vi "Server send.vi"() -> ()   [LabVIEW 2016, in "数据传输系统-03.lvlib" / "自动更新.lvlib" / "TCP文件传输系统.lvlib"]
uses:
  <vilib>/Utility/miscctls.llb/LVPointTypeDef.ctl
  <vilib>/Utility/sysdir.llb/System Directory Type.ctl
  <vilib>/Averna/Notify Icon/NotifyIcon.llb/BalloonIcon.ctl
  <vilib>/Averna/Notify Icon/NotifyIcon.llb/GetSelectedItemEvent.vi
  <vilib>/Averna/Notify Icon/NotifyIcon.llb/SetVisible.vi
  <vilib>/Averna/Notify Icon/NotifyIcon.llb/SetMenuDefaultItem.vi
  <vilib>/Averna/Notify Icon/NotifyIcon.llb/SetTipText.vi
  <vilib>/Averna/Notify Icon/NotifyIcon.llb/NotifyIcon.lvclass
panel:
  in  "选项卡控件 2":enum32{"数据传输系统", "固定站系统", "环保认证"}(tab)
  in  "选项卡控件":T1(tab)
  out "TCP发送全局簇":T2
  out "文件传输的路径":path
  in  "Application":string="版本升级文档.txt"
  in  "远程端口或服务名称":u16=11235
  out "本机网络地址":string="192.168.1.250"
  out "TCP发送全局簇 2":T2
  out "文件传输的路径 2":path
  in  "Application 2":string="update.exe"
  in  "远程端口或服务名称 2":u16=11236
  out "本机网络地址 2":string="192.168.1.250"
  out "TCP发送全局簇 3":T2
  out "文件传输的路径 3":path
  in  "Application 3":string="平台数据传输系统.exe"
  in  "远程端口或服务名称 3":u16=11234
  out "本机网络地址 3":string="192.168.1.250"
  in  "选项卡控件 3":enum32{"固定站版本txt", "固定站update", "固定站exe"}(tab)
  in  "Application 5":string="版本升级文档.txt"
  out "TCP发送全局簇 5":T2
  out "本机网络地址 5":string="192.168.1.250"
  in  "远程端口或服务名称 5":u16=10051
  out "文件传输的路径 5":path
  out "文件传输的路径 6":path
  in  "远程端口或服务名称 6":u16=10052
  out "本机网络地址 6":string="192.168.1.250"
  out "TCP发送全局簇 6":T2
  in  "Application 6":string="update.exe"
  in  "Application 4":string="一体化水质自动监测系统.exe"
  out "TCP发送全局簇 4":T2
  out "本机网络地址 4":string="192.168.1.250"
  in  "远程端口或服务名称 4":u16=10050
  out "文件传输的路径 4":path
  in  "选项卡控件 4":enum32{"环保认证版本txt", "环保认证update", "环保认证exe"}(tab)
  in  "Application 7":string="版本升级文档.txt"
  out "TCP发送全局簇 7":T2
  out "本机网络地址 7":string="192.168.1.250"
  in  "远程端口或服务名称 7":u16=10061
  out "文件传输的路径 7":path
  out "文件传输的路径 8":path
  in  "远程端口或服务名称 8":u16=10062
  out "本机网络地址 8":string="192.168.1.250"
  out "TCP发送全局簇 8":T2
  in  "Application 8":string="update.exe"
  in  "Application 9":string="一体化微型水质监测站.exe"
  out "TCP发送全局簇 9":T2
  out "本机网络地址 9":string="192.168.1.250"
  in  "远程端口或服务名称 9":u16=10050
  out "文件传输的路径 9":path
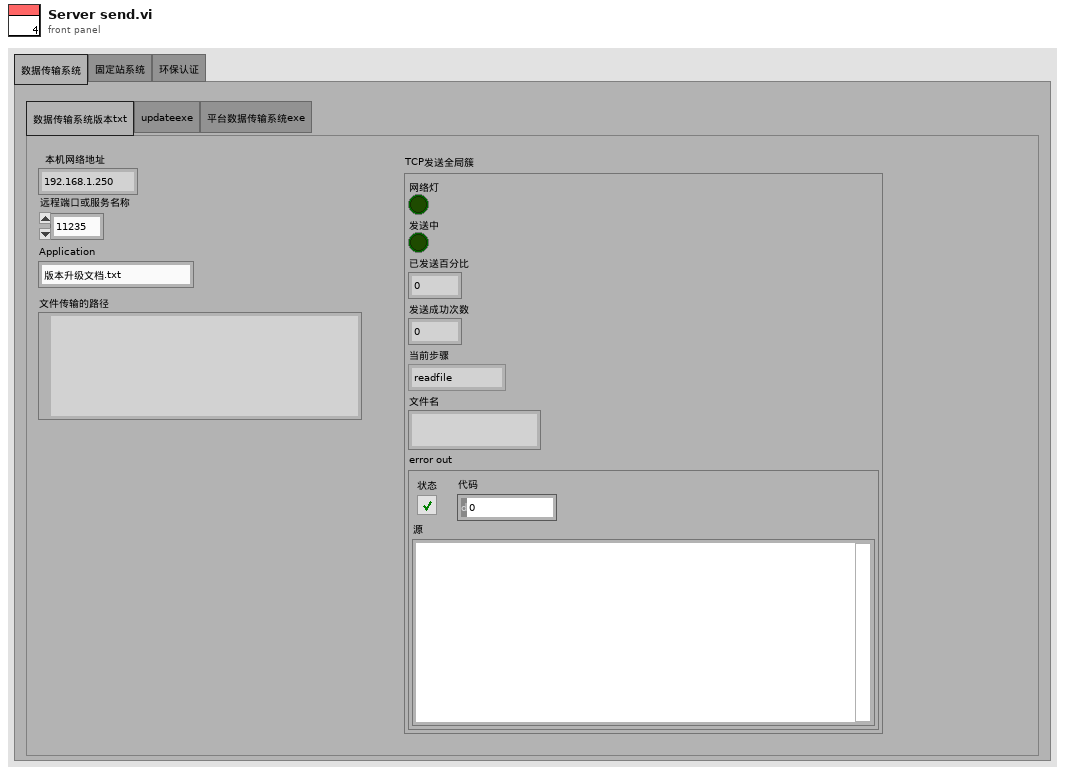
[diagram p1: front panel]
types:
  T1 = enum32{"数据传输系统版本txt", "updateexe", "平台数据传输系统exe"}
  T2 = cluster{"网络灯":bool, "发送中":bool, "已发送百分比":u8, "发送成功次数":dbl, "当前步骤":enum16{"readfile", "init", "sendhead", "sendcontent", "sendsuccess", "over"}, "文件名":string, "error out":errorcluster}
  T3 = enum32{"Invalid", "Standard", "Closed", "Hidden", "Minimized", "Maximized"}
  T4 = typedef "LVPointTypeDef.ctl" = cluster{"Horizontal":i16, "Vertical":i16}
  T5 = typedef "NotifyIcon.lvlib/NotifyIcon.lvclass/BalloonIcon.ctl" = enum32{"None", "Information", "Warning", "Error"}
  T6 = typedef "System Directory Type.ctl" = i32
  T7 = enum32{"invalid app kind", "Development System", "Run Time System", "Student Edition", "Embedded LabVIEW", "Evaluation", "Custom"}
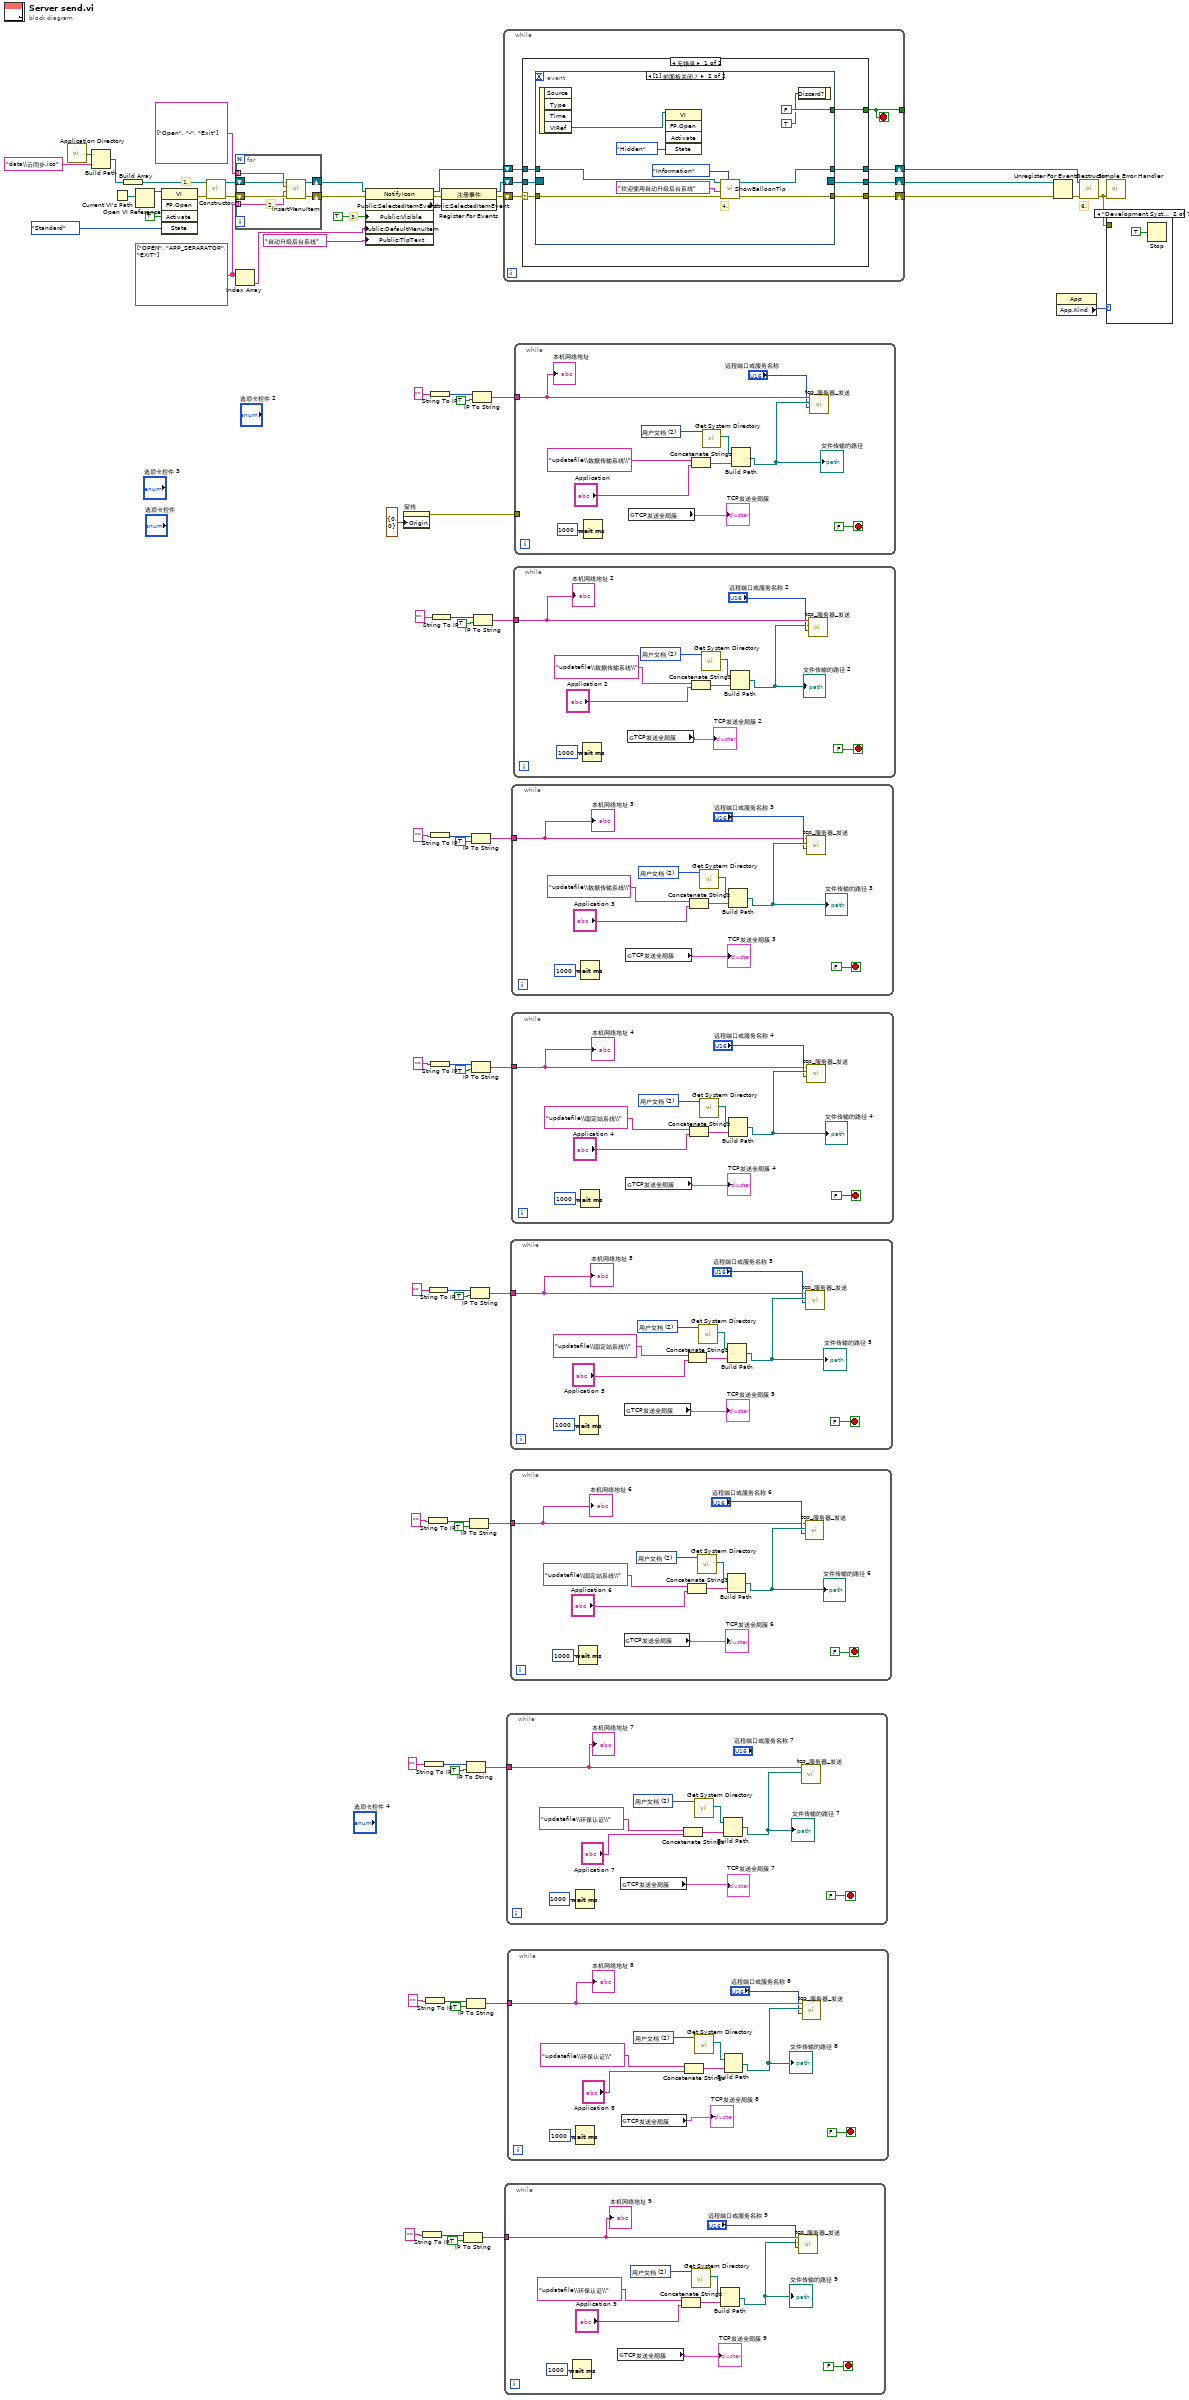
[diagram p0: block diagram]
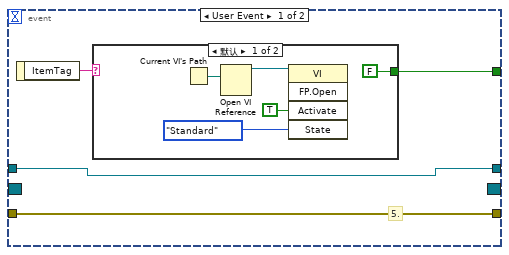
[diagram p2: hidden frame]
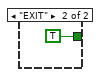
[diagram p3: hidden frame]
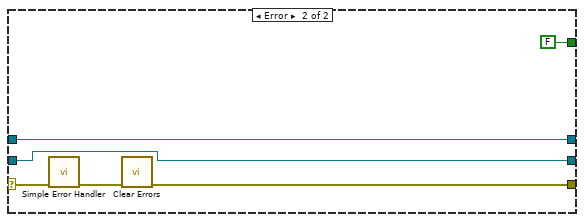
[diagram p4: hidden frame]
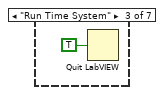
[diagram p6: hidden frame]
diagram:
  w37 = string[] ["OPEN", "APP_SEPARATOR", "EXIT"]
  # "6."
  # "3."
  # "1."
  n1 = call <vilib>:"Application Directory.vi"() -> ("Application Directory"=w35:path)
  n2 = Build Path(base path=w35, name or relative path="data\\云同步.ico" ("名称或相对路径")) -> (appended path=w45:path)
  n3 = Current VI's Path() -> (path=w32:path)
  n4 = Build Array(w45) -> (w40:path[])
  n5 = Open VI Reference(vi path=w32) -> (vi reference=w31:refnum<vi>)  [unwired: 5 in, 1 out]
  n6 = invoke class="VI" method="FP.Open"(reference=w31, "Activate"=TRUE ("激活？"), "State"=T3."Standard" ("状态")) -> (error out=w30:errorcluster)  [unwired: 2 in, 4 out]
  n7 = call <vilib>:"Constructor.vi"("error in"=w30, "IconFilePathList"=w40) -> ("error out"=w44:errorcluster, "NotifyIcon"=w36:refnum<class "NotifyIcon.lvclass">)  [unwired: 8 in]
  n8 = for {
    shift-right: [w72] -> w55
    shift-left: w44 -> [w73]
    tunnel: string[] ["Open", "-", "Exit"] -> [w71] mode=indexing
    tunnel: w37 -> [w70] mode=indexing
    shift-right: [w68] -> w54
    shift-left: w36 -> [w69]
    # "2."
    n9 = call <vilib>:"InsertMenuItem.vi"("error in"=w73, "ItemTag"=w70, "ItemName"=w71, "NotifyIcon in"=w69) -> ("error out"=w72:errorcluster, "NotifyIcon out"=w68:refnum<class "NotifyIcon.lvclass">)  [unwired: 6 in]
  }
  n10 = Index Array(array=w37) -> (element=w38:string)  [unwired: 1 in]
  n11 = property class="NotifyIcon"(reference=w54, error in=w55, "Public:Visible"=TRUE ("Visible"), "Public:DefaultMenuItem"=w38, "Public:TipText"="自动升级后台系统" ("TipText")) -> (reference out=w51:refnum<class "NotifyIcon.lvclass">, error out=w43:errorcluster, "Public:SelectedItemEvent"=w42:refnum<user-event>)
  n12 = property on="窗格" class="Pane"("Origin"=T4 {"Horizontal"=0, "Vertical"=0} ("原点")) -> (error out=w25:errorcluster)  [unwired: 2 in, 1 out]
  n13 = String To IP(1:"" ("名称")) -> (0:w2:u32)
  n14 = String To IP(1:"" ("名称")) -> (0:w10:u32)
  n15 = String To IP(1:"" ("名称")) -> (0:w6:u32)
  n16 = String To IP(1:"" ("名称")) -> (0:w14:u32)
  n17 = String To IP(1:"" ("名称")) -> (0:w19:u32)
  n18 = String To IP(1:"" ("名称")) -> (0:w58:u32)
  n19 = String To IP(1:"" ("名称")) -> (0:w22:u32)
  n20 = String To IP(1:"" ("名称")) -> (0:w65:u32)
  n21 = String To IP(1:"" ("名称")) -> (0:w61:u32)
  n22 = register-events(error in=w43, w42) -> (reference out=w27:refnum<event-registration>, error out=w28:errorcluster)  [unwired: 1 in]
  n23 = IP To String(1:TRUE ("句点符号？(F)"), 2:w2) -> (0:w1:string)
  n24 = IP To String(1:TRUE ("句点符号？(F)"), 2:w10) -> (0:w9:string)
  n25 = IP To String(1:TRUE ("句点符号？(F)"), 2:w6) -> (0:w5:string)
  n26 = IP To String(1:TRUE ("句点符号？(F)"), 2:w14) -> (0:w13:string)
  n27 = IP To String(1:TRUE ("句点符号？(F)"), 2:w19) -> (0:w20:string)
  n28 = IP To String(1:TRUE ("句点符号？(F)"), 2:w58) -> (0:w59:string)
  n29 = IP To String(1:TRUE ("句点符号？(F)"), 2:w22) -> (0:w21:string)
  n30 = IP To String(1:TRUE ("句点符号？(F)"), 2:w65) -> (0:w64:string)
  n31 = IP To String(1:TRUE ("句点符号？(F)"), 2:w61) -> (0:w60:string)
  n32 = while {
    shift-right: [w77] -> w49
    shift-left: w28 -> [w76]
    shift-right: [w78] -> w47
    shift-left: w51 -> [w79]
    shift-right: [w75] -> w48
    shift-left: w27 -> [w80]
    tunnel: [w74] -> _
    stop <- w74 stop-if-true
    n33 = case shown="无错误" w76 {
      selector: w76 -> [w82 w113]
      tunnel: w80 -> [w87 w108]
      tunnel: w79 -> [w86 w109]
      tunnel: [w85 w109] -> w78
      tunnel: [w84 w111] -> w77
      tunnel: [w83 FALSE ("Discard?")] -> w74
      tunnel: [w81 w108] -> w75
      frame No Error {
        n34 = event shown="[1] 前面板关闭？" {
          selector: w87 -> [_ _]
          dyn-events: [_ _] -> w81
          timeout: _ -> [_ _]
          tunnel: w82 -> [w90 w106]
          tunnel: [w90 w105] -> w84
          tunnel: [w89 FALSE ("Discard?")] -> w83
          tunnel: w86 -> [w88 w107]
          tunnel: [w88 w104] -> w85
          event User Event {
            # "5."
            n35 = event-data() -> ("ItemTag"=w91:string)  [unwired: 1 in]
            n36 = case shown="默认" w91 {
              tunnel: [FALSE TRUE] -> w89
              frame Default {
                n37 = Current VI's Path() -> (path=w93:path)
                n38 = Open VI Reference(vi path=w93) -> (vi reference=w94:refnum<vi>)  [unwired: 5 in, 1 out]
                n39 = invoke class="VI" method="FP.Open"(reference=w94, "Activate"=TRUE ("激活？"), "State"=T3."Standard" ("状态")) -> ()  [unwired: 2 in, 5 out]
              }
              frame "EXIT" {
              }
            }
          }
          event Panel Close? {
            # "4."
            n40 = event-data() -> ("VIRef"=w100:refnum<vi>)  [unwired: 1 in, 3 out]
            n41 = invoke class="VI" method="FP.Open"(reference=w100, "State"=T3."Hidden" ("状态")) -> ()  [unwired: 3 in, 5 out]
            n42 = call <vilib>:"ShowBalloonTip.vi"("Balloon Icon"=BalloonIcon."Information", "error in"=w106, "Text"="欢迎使用自动升级后台系统", "NotifyIcon in"=w107) -> ("error out"=w105:errorcluster, "NotifyIcon out"=w104:refnum<class "NotifyIcon.lvclass">)  [unwired: 6 in]
            n43 = event-data("Discard?"=TRUE ("放弃？")) -> ()  [unwired: 1 in, 1 out]
          }
        }
      }
      frame Error {
        n44 = call <vilib>:"Simple Error Handler.vi"("error in (no error)"=w113) -> ("error out"=w112:errorcluster)  [unwired: 4 in, 4 out]
        n45 = call <vilib>:"Clear Errors.vi"("error in (no error)"=w112) -> ("error out"=w111:errorcluster)  [unwired: 5 in, 1 out]
      }
    }
  }
  n46 = while {
    tunnel: w1 -> [w118]
    stop <- FALSE stop-if-true
    w123 = T6 2 items=["用户目录"=0, "用户桌面"=1, "用户文档"=2, "用户应用程序数据"=3, "用户设置"=4, "用户临时目录"=5, "公共文档"=6, "公共应用程序数据"=7, "公共设置"=8, "公共缓存"=13, "系统核心库"=9, "系统安装库"=10, "应用程序文件"=11, "启动盘根目录"=12] ("system directory type")
    n47 = Wait (ms)(milliseconds to wait=u32 1000 ("等待时间（毫秒）")) -> ()  [unwired: 1 out]
    n48 = global read "全局变量1.vi" "TCP发送全局簇"() -> (→"TCP发送全局簇 9":T2)
    n49 = Concatenate Strings("updatefile\\环保认证\\" ("condition"), "Application 9") -> (w122:string)
    n50 = call <vilib>:"Get System Directory.vi"("system directory type"=w123) -> ("system directory"=w121:path)  [unwired: 10 in]
    n51 = Build Path(base path=w121, name or relative path=w122) -> (appended path=w114:path)
    "文件传输的路径 9" <- w114
    n52 = call "tcp_服务器_发送.vi"("远程端口或服务名称"="远程端口或服务名称 9", "原文件路径（使用对话框）"=w114, "服务器网络地址"=w118) -> ()  [unwired: 9 in]
    "本机网络地址 9" <- w118
  }
  n53 = while {
    tunnel: w9 -> [w128]
    stop <- FALSE stop-if-true
    w133 = T6 2 items=["用户目录"=0, "用户桌面"=1, "用户文档"=2, "用户应用程序数据"=3, "用户设置"=4, "用户临时目录"=5, "公共文档"=6, "公共应用程序数据"=7, "公共设置"=8, "公共缓存"=13, "系统核心库"=9, "系统安装库"=10, "应用程序文件"=11, "启动盘根目录"=12] ("system directory type")
    n54 = Wait (ms)(milliseconds to wait=u32 1000 ("等待时间（毫秒）")) -> ()  [unwired: 1 out]
    n55 = global read "全局变量1.vi" "TCP发送全局簇"() -> (→"TCP发送全局簇 7":T2)
    n56 = Concatenate Strings("updatefile\\环保认证\\" ("condition"), "Application 7") -> (w132:string)
    n57 = call <vilib>:"Get System Directory.vi"("system directory type"=w133) -> ("system directory"=w131:path)  [unwired: 10 in]
    n58 = Build Path(base path=w131, name or relative path=w132) -> (appended path=w126:path)
    "文件传输的路径 7" <- w126
    n59 = call "tcp_服务器_发送.vi"("原文件路径（使用对话框）"=w126, "服务器网络地址"=w128) -> ()  [unwired: 10 in]
    "本机网络地址 7" <- w128
  }
  n60 = while {
    tunnel: w5 -> [w139]
    stop <- FALSE stop-if-true
    w144 = T6 2 items=["用户目录"=0, "用户桌面"=1, "用户文档"=2, "用户应用程序数据"=3, "用户设置"=4, "用户临时目录"=5, "公共文档"=6, "公共应用程序数据"=7, "公共设置"=8, "公共缓存"=13, "系统核心库"=9, "系统安装库"=10, "应用程序文件"=11, "启动盘根目录"=12] ("system directory type")
    n61 = Wait (ms)(milliseconds to wait=u32 1000 ("等待时间（毫秒）")) -> ()  [unwired: 1 out]
    n62 = global read "全局变量1.vi" "TCP发送全局簇"() -> (→"TCP发送全局簇 8":T2)
    n63 = Concatenate Strings("updatefile\\环保认证\\" ("condition"), "Application 8") -> (w143:string)
    n64 = call <vilib>:"Get System Directory.vi"("system directory type"=w144) -> ("system directory"=w142:path)  [unwired: 10 in]
    n65 = Build Path(base path=w142, name or relative path=w143) -> (appended path=w136:path)
    "文件传输的路径 8" <- w136
    n66 = call "tcp_服务器_发送.vi"("远程端口或服务名称"="远程端口或服务名称 8", "原文件路径（使用对话框）"=w136, "服务器网络地址"=w139) -> ()  [unwired: 9 in]
    "本机网络地址 8" <- w139
  }
  n67 = while {
    tunnel: w13 -> [w149]
    stop <- FALSE stop-if-true
    w155 = T6 2 items=["用户目录"=0, "用户桌面"=1, "用户文档"=2, "用户应用程序数据"=3, "用户设置"=4, "用户临时目录"=5, "公共文档"=6, "公共应用程序数据"=7, "公共设置"=8, "公共缓存"=13, "系统核心库"=9, "系统安装库"=10, "应用程序文件"=11, "启动盘根目录"=12] ("system directory type")
    n68 = Wait (ms)(milliseconds to wait=u32 1000 ("等待时间（毫秒）")) -> ()  [unwired: 1 out]
    n69 = global read "全局变量1.vi" "TCP发送全局簇"() -> (→"TCP发送全局簇 6":T2)
    n70 = Concatenate Strings("updatefile\\固定站系统\\" ("condition"), "Application 6") -> (w154:string)
    n71 = call <vilib>:"Get System Directory.vi"("system directory type"=w155) -> ("system directory"=w153:path)  [unwired: 10 in]
    n72 = Build Path(base path=w153, name or relative path=w154) -> (appended path=w151:path)
    "文件传输的路径 6" <- w151
    n73 = call "tcp_服务器_发送.vi"("远程端口或服务名称"="远程端口或服务名称 6", "原文件路径（使用对话框）"=w151, "服务器网络地址"=w149) -> ()  [unwired: 9 in]
    "本机网络地址 6" <- w149
  }
  n74 = while {
    tunnel: w20 -> [w160]
    stop <- FALSE stop-if-true
    w166 = T6 2 items=["用户目录"=0, "用户桌面"=1, "用户文档"=2, "用户应用程序数据"=3, "用户设置"=4, "用户临时目录"=5, "公共文档"=6, "公共应用程序数据"=7, "公共设置"=8, "公共缓存"=13, "系统核心库"=9, "系统安装库"=10, "应用程序文件"=11, "启动盘根目录"=12] ("system directory type")
    n75 = Wait (ms)(milliseconds to wait=u32 1000 ("等待时间（毫秒）")) -> ()  [unwired: 1 out]
    n76 = global read "全局变量1.vi" "TCP发送全局簇"() -> (→"TCP发送全局簇 5":T2)
    n77 = Concatenate Strings("updatefile\\固定站系统\\" ("condition"), "Application 5") -> (w165:string)
    n78 = call <vilib>:"Get System Directory.vi"("system directory type"=w166) -> ("system directory"=w164:path)  [unwired: 10 in]
    n79 = Build Path(base path=w164, name or relative path=w165) -> (appended path=w162:path)
    "文件传输的路径 5" <- w162
    n80 = call "tcp_服务器_发送.vi"("远程端口或服务名称"="远程端口或服务名称 5", "原文件路径（使用对话框）"=w162, "服务器网络地址"=w160) -> ()  [unwired: 9 in]
    "本机网络地址 5" <- w160
  }
  n81 = while {
    tunnel: w59 -> [w171]
    stop <- FALSE stop-if-true
    w177 = T6 2 items=["用户目录"=0, "用户桌面"=1, "用户文档"=2, "用户应用程序数据"=3, "用户设置"=4, "用户临时目录"=5, "公共文档"=6, "公共应用程序数据"=7, "公共设置"=8, "公共缓存"=13, "系统核心库"=9, "系统安装库"=10, "应用程序文件"=11, "启动盘根目录"=12] ("system directory type")
    n82 = Wait (ms)(milliseconds to wait=u32 1000 ("等待时间（毫秒）")) -> ()  [unwired: 1 out]
    n83 = global read "全局变量1.vi" "TCP发送全局簇"() -> (→"TCP发送全局簇 3":T2)
    n84 = Concatenate Strings("updatefile\\数据传输系统\\" ("condition"), "Application 3") -> (w176:string)
    n85 = call <vilib>:"Get System Directory.vi"("system directory type"=w177) -> ("system directory"=w175:path)  [unwired: 10 in]
    n86 = Build Path(base path=w175, name or relative path=w176) -> (appended path=w173:path)
    "文件传输的路径 3" <- w173
    n87 = call "tcp_服务器_发送.vi"("远程端口或服务名称"="远程端口或服务名称 3", "原文件路径（使用对话框）"=w173, "服务器网络地址"=w171) -> ()  [unwired: 9 in]
    "本机网络地址 3" <- w171
  }
  n88 = while {
    tunnel: w21 -> [w182]
    stop <- FALSE stop-if-true
    w188 = T6 2 items=["用户目录"=0, "用户桌面"=1, "用户文档"=2, "用户应用程序数据"=3, "用户设置"=4, "用户临时目录"=5, "公共文档"=6, "公共应用程序数据"=7, "公共设置"=8, "公共缓存"=13, "系统核心库"=9, "系统安装库"=10, "应用程序文件"=11, "启动盘根目录"=12] ("system directory type")
    n89 = Wait (ms)(milliseconds to wait=u32 1000 ("等待时间（毫秒）")) -> ()  [unwired: 1 out]
    n90 = global read "全局变量1.vi" "TCP发送全局簇"() -> (→"TCP发送全局簇 4":T2)
    n91 = Concatenate Strings("updatefile\\固定站系统\\" ("condition"), "Application 4") -> (w187:string)
    n92 = call <vilib>:"Get System Directory.vi"("system directory type"=w188) -> ("system directory"=w186:path)  [unwired: 10 in]
    n93 = Build Path(base path=w186, name or relative path=w187) -> (appended path=w184:path)
    "文件传输的路径 4" <- w184
    n94 = call "tcp_服务器_发送.vi"("远程端口或服务名称"="远程端口或服务名称 4", "原文件路径（使用对话框）"=w184, "服务器网络地址"=w182) -> ()  [unwired: 9 in]
    "本机网络地址 4" <- w182
  }
  n95 = while {
    tunnel: w60 -> [w195]
    stop <- FALSE stop-if-true
    w199 = T6 2 items=["用户目录"=0, "用户桌面"=1, "用户文档"=2, "用户应用程序数据"=3, "用户设置"=4, "用户临时目录"=5, "公共文档"=6, "公共应用程序数据"=7, "公共设置"=8, "公共缓存"=13, "系统核心库"=9, "系统安装库"=10, "应用程序文件"=11, "启动盘根目录"=12] ("system directory type")
    n96 = Wait (ms)(milliseconds to wait=u32 1000 ("等待时间（毫秒）")) -> ()  [unwired: 1 out]
    n97 = global read "全局变量1.vi" "TCP发送全局簇"() -> (→"TCP发送全局簇 2":T2)
    n98 = Concatenate Strings("updatefile\\数据传输系统\\" ("condition"), "Application 2") -> (w198:string)
    n99 = call <vilib>:"Get System Directory.vi"("system directory type"=w199) -> ("system directory"=w197:path)  [unwired: 10 in]
    n100 = Build Path(base path=w197, name or relative path=w198) -> (appended path=w191:path)
    "文件传输的路径 2" <- w191
    n101 = call "tcp_服务器_发送.vi"("远程端口或服务名称"="远程端口或服务名称 2", "原文件路径（使用对话框）"=w191, "服务器网络地址"=w195) -> ()  [unwired: 9 in]
    "本机网络地址 2" <- w195
  }
  n102 = while {
    tunnel: w64 -> [w209]
    tunnel: w25 -> [_]
    stop <- FALSE stop-if-true
    w210 = T6 2 items=["用户目录"=0, "用户桌面"=1, "用户文档"=2, "用户应用程序数据"=3, "用户设置"=4, "用户临时目录"=5, "公共文档"=6, "公共应用程序数据"=7, "公共设置"=8, "公共缓存"=13, "系统核心库"=9, "系统安装库"=10, "应用程序文件"=11, "启动盘根目录"=12] ("system directory type")
    n103 = Wait (ms)(milliseconds to wait=u32 1000 ("等待时间（毫秒）")) -> ()  [unwired: 1 out]
    n104 = global read "全局变量1.vi" "TCP发送全局簇"() -> (→"TCP发送全局簇":T2)
    n105 = Concatenate Strings("updatefile\\数据传输系统\\" ("condition"), "Application") -> (w208:string)
    n106 = call <vilib>:"Get System Directory.vi"("system directory type"=w210) -> ("system directory"=w206:path)  [unwired: 10 in]
    n107 = Build Path(base path=w206, name or relative path=w208) -> (appended path=w205:path)
    "文件传输的路径" <- w205
    n108 = call "tcp_服务器_发送.vi"("远程端口或服务名称"="远程端口或服务名称", "原文件路径（使用对话框）"=w205, "服务器网络地址"=w209) -> ()  [unwired: 9 in]
    "本机网络地址" <- w209
  }
  n109 = Unregister For Events(event registration refnum=w48, error in=w49) -> (error out=w50:errorcluster)
  n110 = property class="App"() -> ("App.Kind"=w29:T7)  [unwired: 2 in, 2 out]
  n111 = call <vilib>:"Destructor.vi"("error in"=w50, "NotifyIcon"=w47) -> ("error out"=w46:errorcluster)  [unwired: 9 in]
  n112 = call <vilib>:"Simple Error Handler.vi"("error in (no error)"=w46) -> ()  [unwired: 4 in, 5 out]
  n113 = case shown="\"Development System\"" w29 {
    tunnel: w46 -> [_ _ _ _ _ _ _]
    frame "invalid app kind", Default {
    }
    frame "Development System" {
      n114 = Stop(stop? (T)=TRUE ("可见")) -> ()
    }
    frame "Run Time System" {
      n115 = Quit LabVIEW(quit? (T)=TRUE ("退出？(T)")) -> ()
    }
    frame "Student Edition" {
    }
    frame "Embedded LabVIEW" {
    }
    frame "Evaluation" {
    }
    frame "Custom" {
    }
  }
